vi "Error Processor.vi"(8 "error in (no error)":errorcluster, 11 "Dummy in":refnum<class "Dummy.lvclass">) -> (0 "error out":errorcluster, 3 "Dummy out":refnum<class "Dummy.lvclass">)   [LabVIEW 2020, in "Dummy.lvlib" / "Dummy.lvclass"]
doc: "Use this VI to process all the error that are solvable inside this specific uService. Whatever is not possible to process, let it leave this VI and it will be processed by the Error Manager of the Distributed System."
uses:
  Dummy.lvclass
  TALOS/TALOS_PPL.lvlibp/Father of all uServices/Father of all uServices/Father of all uServices.lvclass
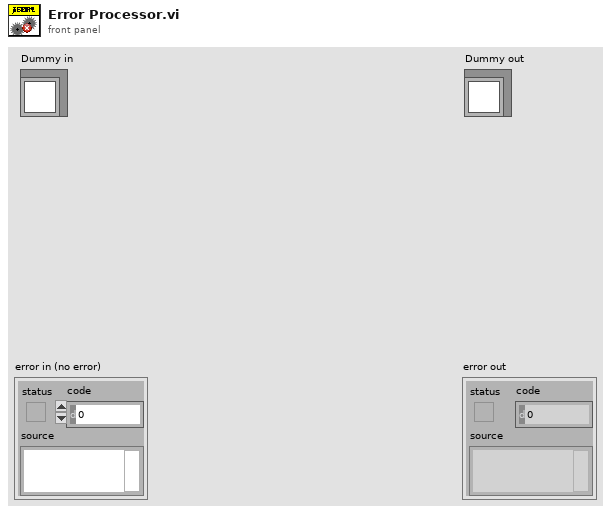
[diagram p1: front panel]
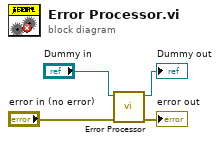
[diagram p0: block diagram]
diagram:
  n1 = call-parent "Error Processor.vi"("error in (no error)"="error in (no error)", "Father of all uServices in"="Dummy in") -> ("error out"=→"error out":errorcluster, "Father of all uServices out"=→"Dummy out":refnum<class "Dummy.lvclass">)  [unwired: 8 in]
